vi "纳清电导率电极校准.vi"() -> ()   [LabVIEW 2016, in "斯坦道多参数.lvlib"]
uses:
  <vilib>/Utility/miscctls.llb/LVPointTypeDef.ctl
  <vilib>/Utility/miscctls.llb/LVPositionTypeDef.ctl
  <vilib>/Analysis/NI_AALBase.lvlib
panel:
  out "当前量程":u16
  out "当前探头类别":string
  out "报警信息":string
  out "温度校准参数":sgl format="%#.2f"
  out "通讯状态":string
  out "第二点校准值":dbl
  out "第一点校准值":dbl
  in  "校准停止":bool
  in  "校准启动":bool
  in  "校准模式":enum16{"单点校准"}(ring)
  out "最小值":sgl format="%#.2f"
  out "最大值":sgl format="%#.2f"
  out "波形图表":sgl(graph) caption="历史曲线"
  out "mean":dbl caption="均值" format="%#.2f"
  out "standard deviation":dbl caption="标准差" format="%#.2f"
  out "变异系数":dbl format="%#.6f"
  out "测量值":sgl format="%#.2f"
  out "提示":string
  out "标液1":sgl
  out "原始光强数值":sgl caption="信号值" format="%#.6f"
  out "温度":dbl format="%#.2f"
  # "电导率电极设定"
  # "℃"
  # "uS/cm"
  # "电阻"
  # "℃"
  # "请选择校准模式:"
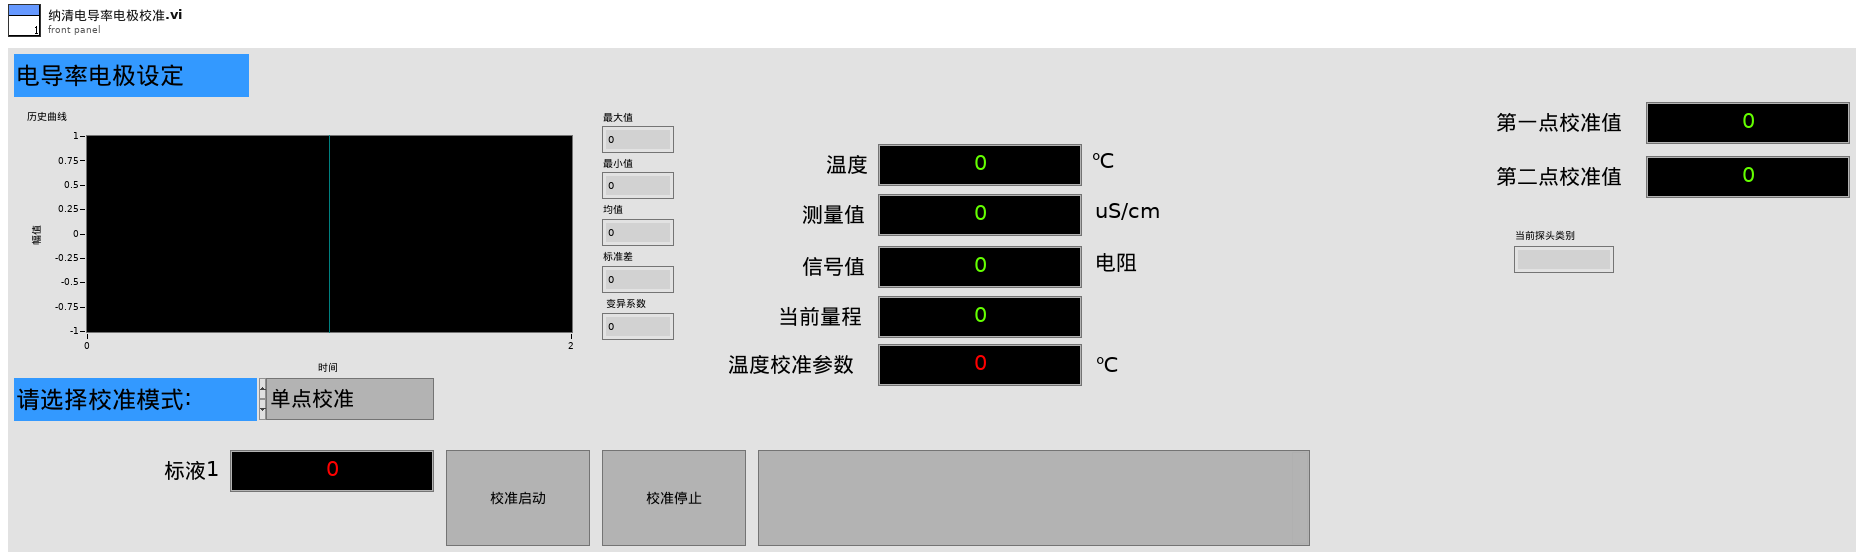
[diagram p1: front panel]
types:
  T1 = typedef "LVPointTypeDef.ctl" = cluster{"Horizontal":i16, "Vertical":i16}
  T2 = typedef "斯坦道多参数.lvlib/校准步骤.ctl" = enum16{"待机", "放置第一点标液", "第一点校准启动", "第一点校准写入", "第一点校准失败", "放置第二点标液", "第二点校准启动", "第二点校准写入", "第二点校准失败", "放置第三点标液", "第三点校准启动", "第三点校准写入", "第三点校准失败", "校准结果写入", "校准结束"}
  T3 = cluster{"报警码":u16, "电导率数据（uS/cm）":sgl, "0x0003 NC":sgl, "温度数据":sgl, "电导率原始信号电阻":sgl, "当前量程":u16, "温度补偿系数":sgl, "0X0009_NC":string, "产品名称":string, "序列号":string, "硬件版本":string, "软件版本":string, "通讯地址":u16, "波特率":u16, "设备类型":u16, "0X0026_NC":string, "第一点原始数据":sgl, "第一点校准数据":sgl, "0X0035_NC":sgl, "0X0037_NC":sgl, "探头校准命令":u16, "温度校准参数":sgl, "温度校准命令":u16}
  T4 = typedef "LVPositionTypeDef.ctl" = cluster{"Left":i32, "Top":i32}
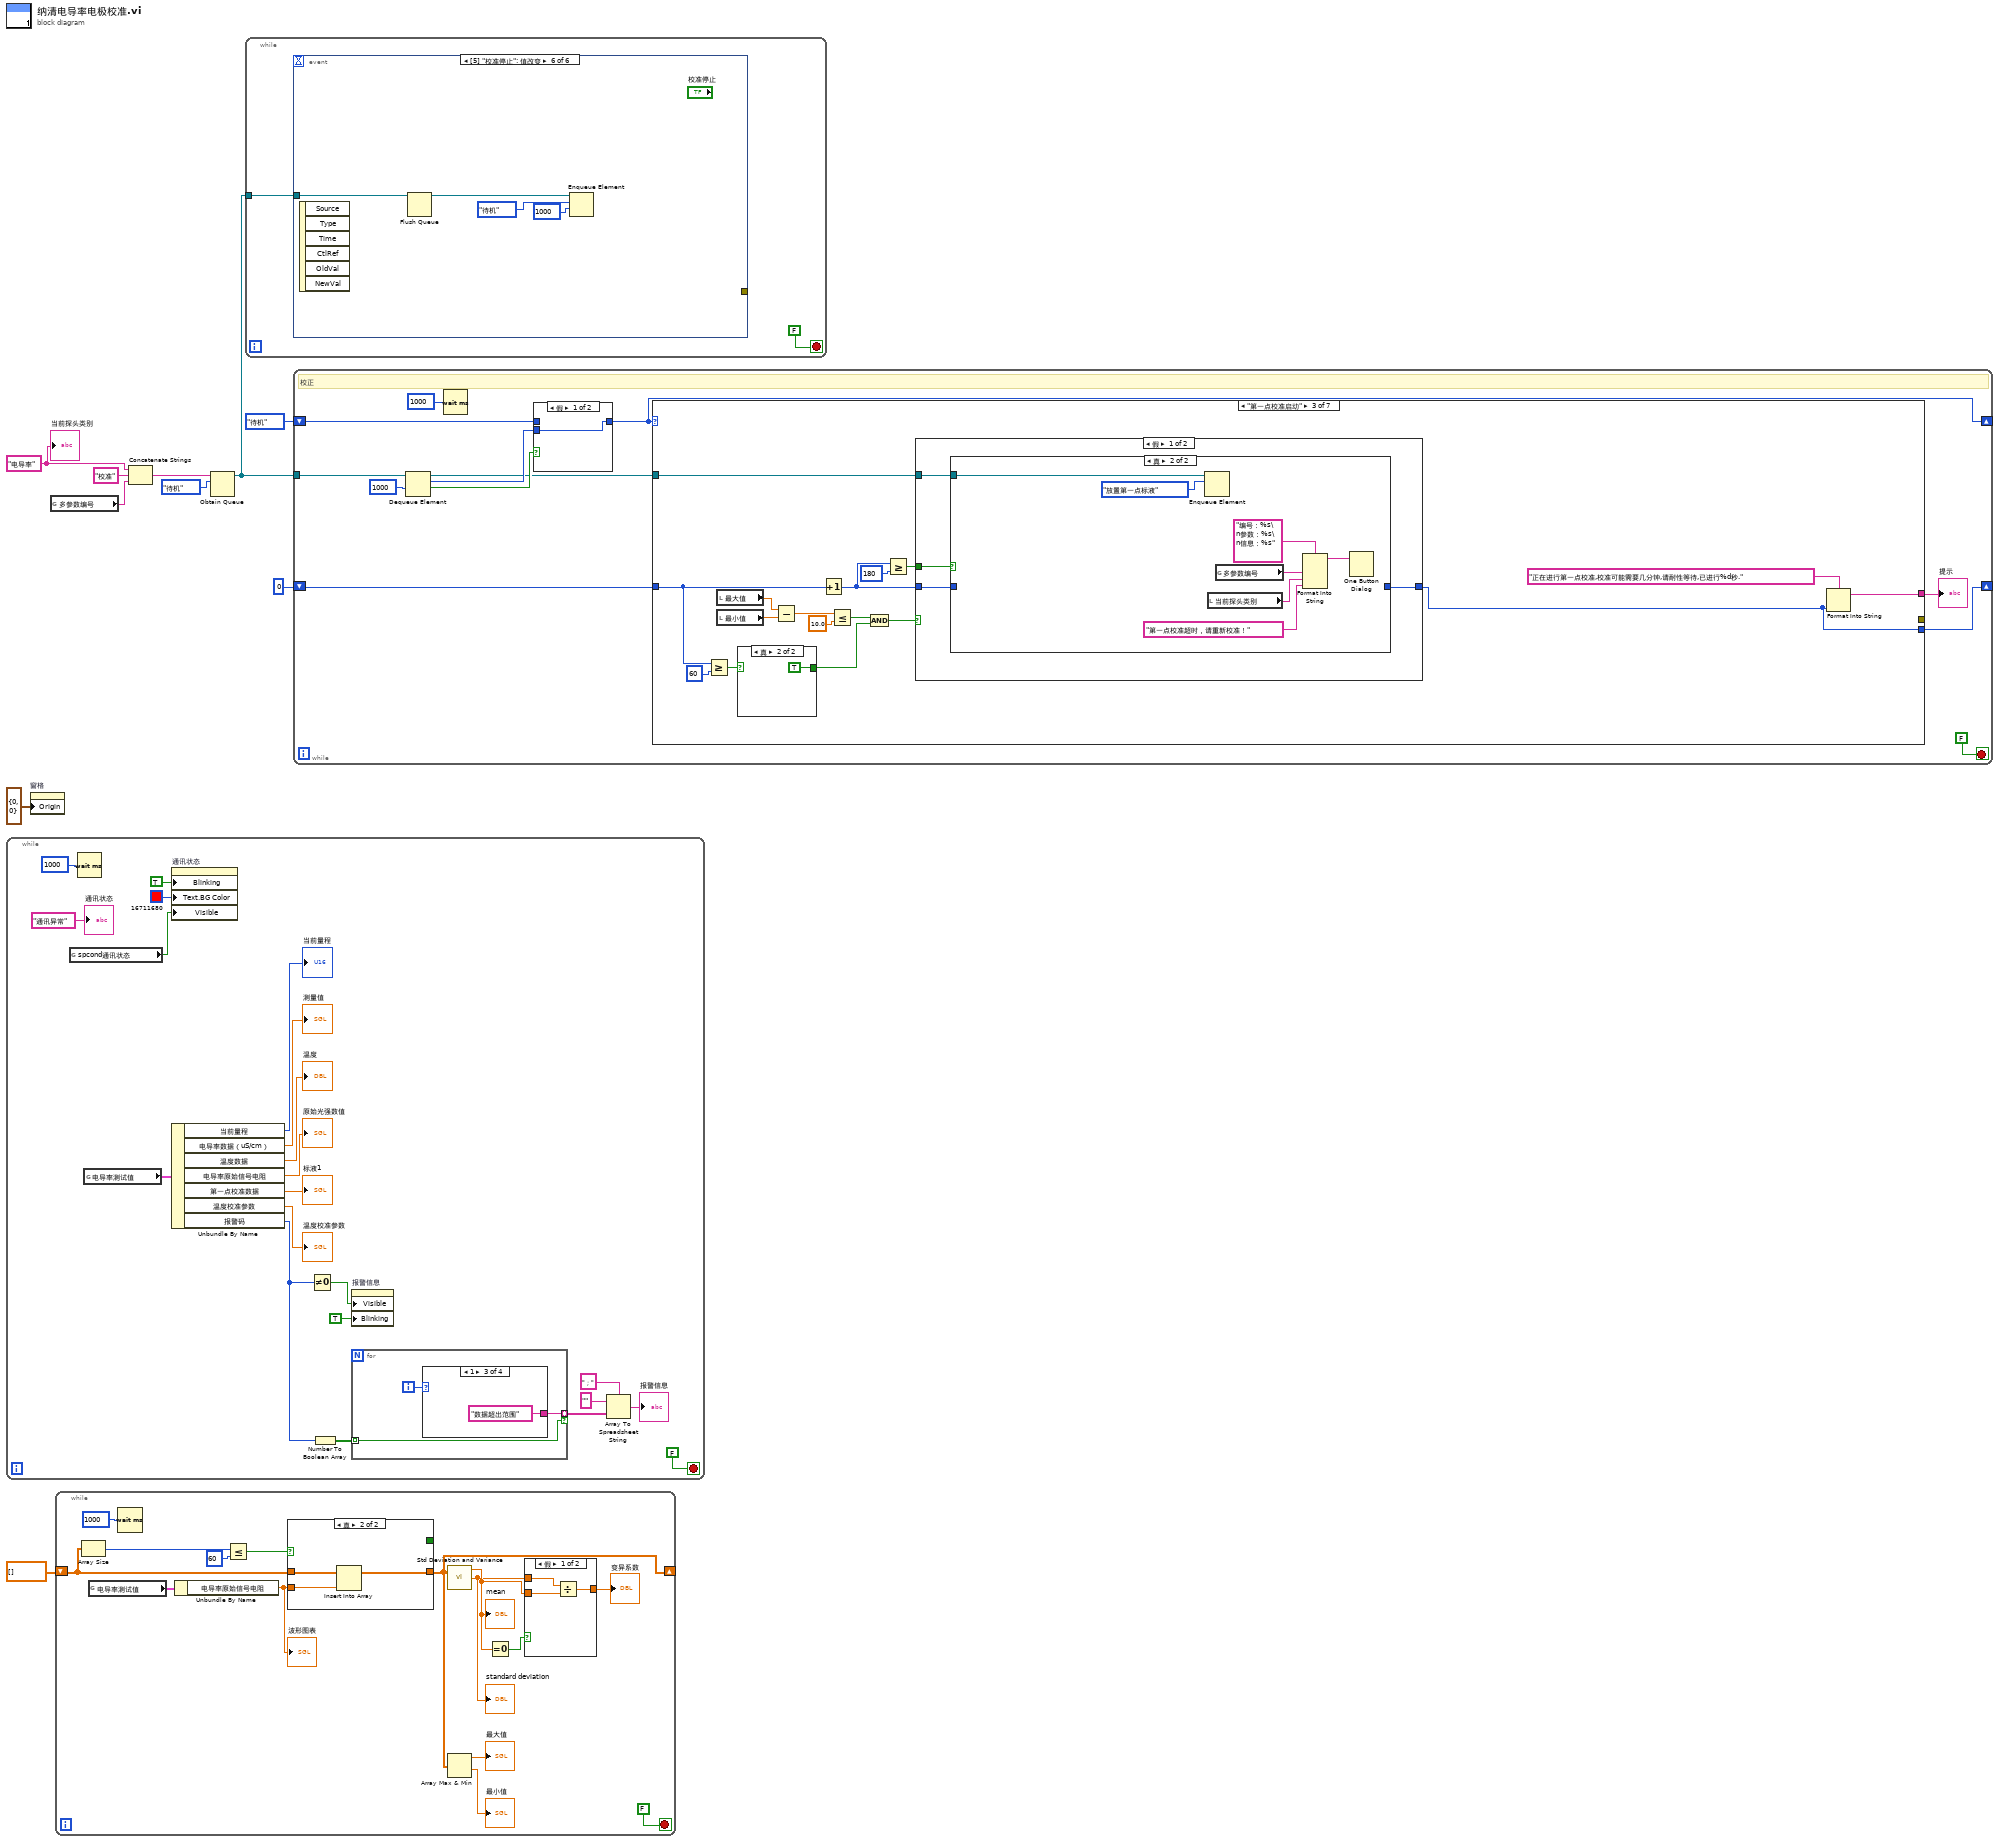
[diagram p0: block diagram]
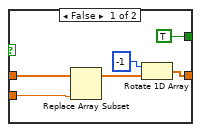
[diagram p3: hidden frame]
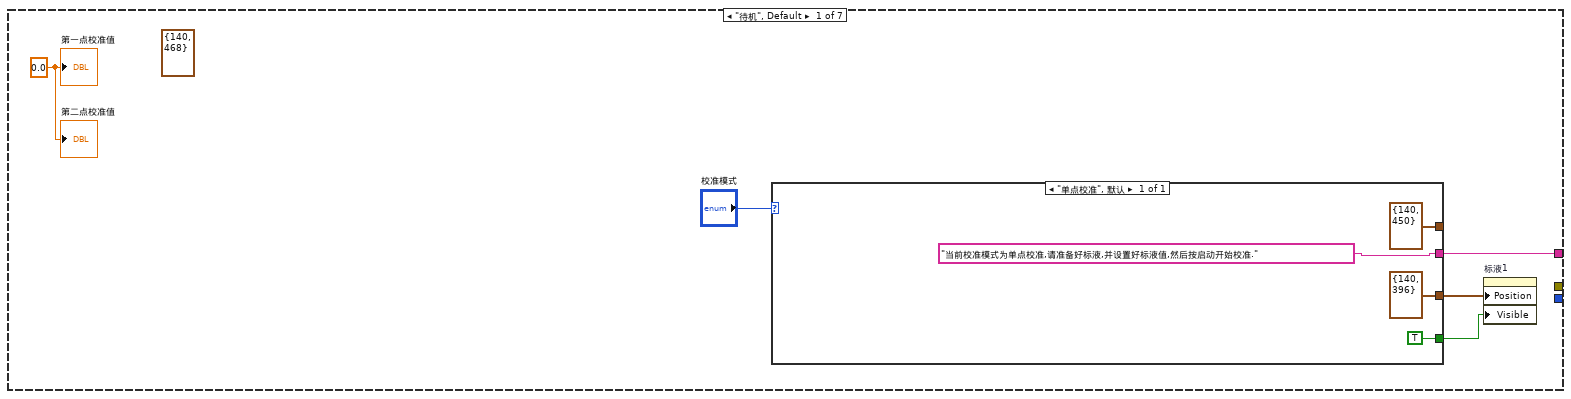
[diagram p5: hidden frame]
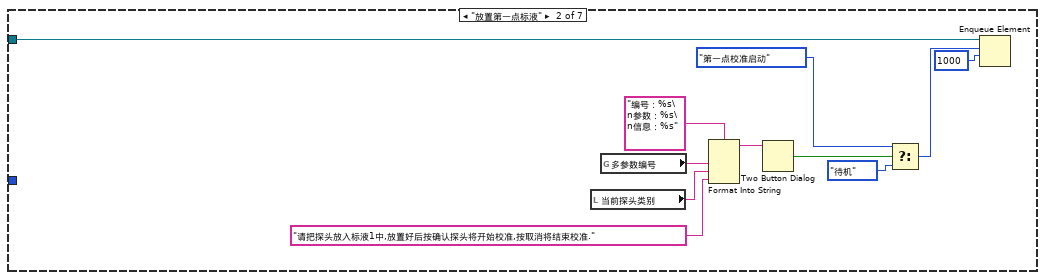
[diagram p6: hidden frame]
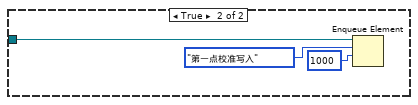
[diagram p8: hidden frame]
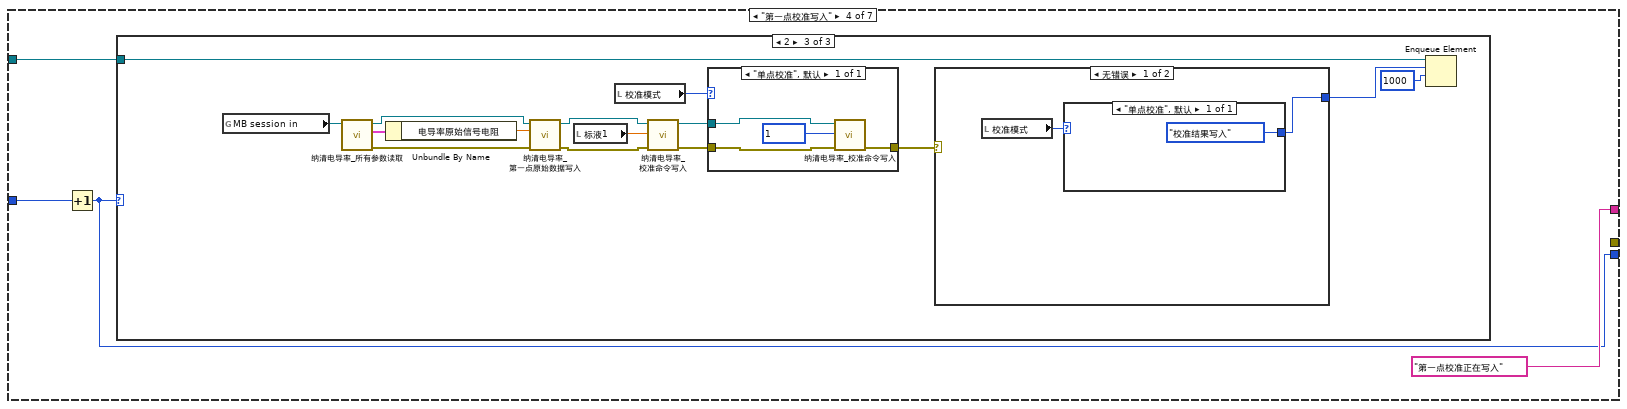
[diagram p10: hidden frame]
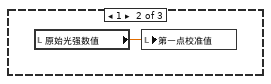
[diagram p12: hidden frame]
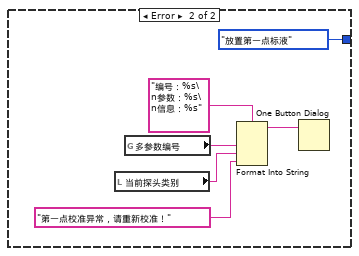
[diagram p13: hidden frame]
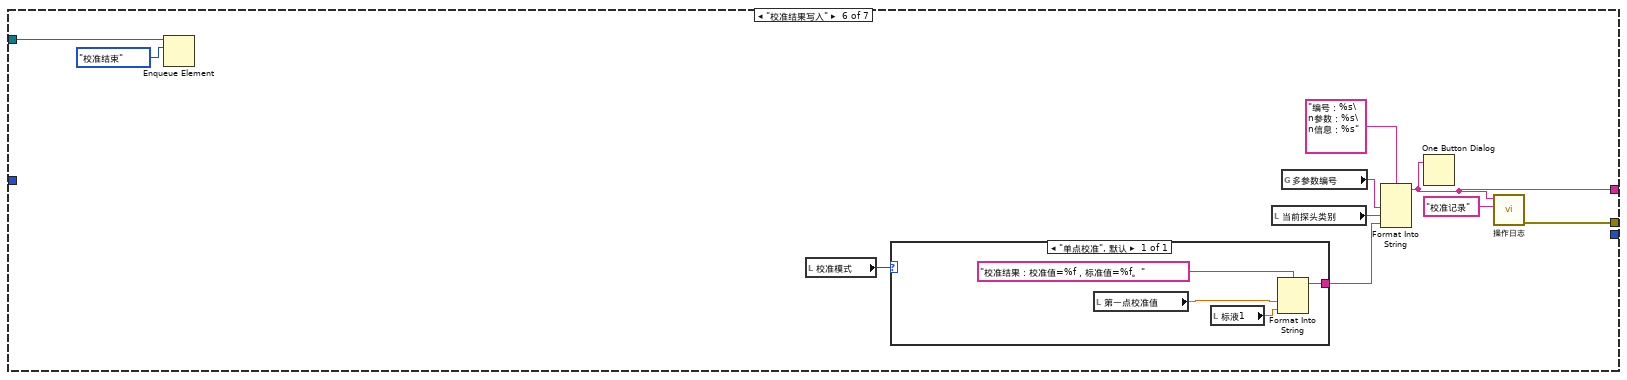
[diagram p15: hidden frame]
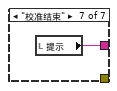
[diagram p16: hidden frame]
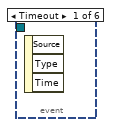
[diagram p17: hidden frame]
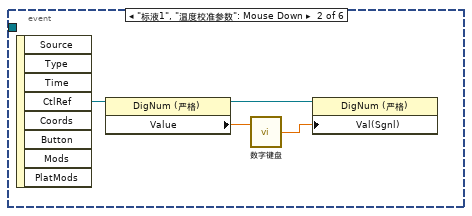
[diagram p18: hidden frame]
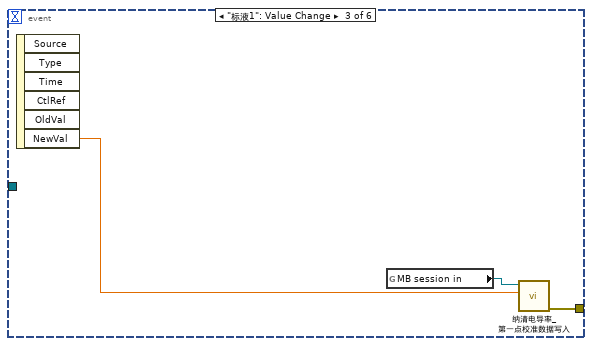
[diagram p19: hidden frame]
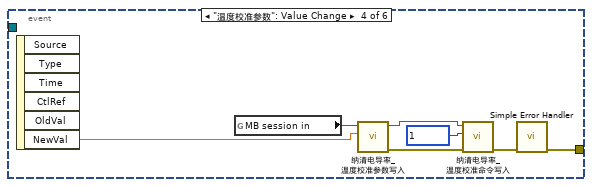
[diagram p20: hidden frame]
diagram:
  w1 = "电导率" ("当前探头类别")
  n1 = while {
    stop <- FALSE stop-if-true
    n2 = global read "多参数全局变量.vi" "spcond通讯状态"() -> (w21:bool)
    n3 = Wait (ms)(milliseconds to wait=u32 1000 ("等待时间（毫秒）")) -> ()  [unwired: 1 out]
    n4 = global read "纳清过程全局变量.vi" "电导率测试值"() -> (w29:T3)
    n5 = property on="通讯状态" class="Str"("Blinking"=TRUE ("闪烁"), "Text.BG Color"=u32 16711680, "Visible"=w21) -> ()  [unwired: 2 in, 2 out]
    n6 = Unbundle By Name(w29) -> ("当前量程"=→"当前量程":u16, "电导率数据（uS/cm）"=→"测量值":sgl, "温度数据"=→"温度":sgl, "电导率原始信号电阻"=→"原始光强数值":sgl, "第一点校准数据"=→"标液1":sgl, "温度校准参数"=→"温度校准参数":sgl, "报警码"=w14:u16)
    n7 = Not Equal To 0?(x=w14) -> (x != 0?=w13:bool)
    n8 = Number To Boolean Array(number=w14) -> (Boolean array=w19:bool[])
    n9 = property on="报警信息" class="Str"("Visible"=w13, "Blinking"=TRUE ("闪烁")) -> ()  [unwired: 2 in, 2 out]
    n10 = for {
      tunnel: w19 -> [w32] mode=indexing
      tunnel: [w33] -> w18 mode=indexing if=w32
      i -> [w34]
      n11 = case shown="1" w34 {
        tunnel: [_ "温度超出范围" "数据超出范围" "温度传感器故障"] -> w33
        frame Default {
        }
        frame 0 {
        }
        frame 1 {
        }
        frame 8 {
        }
      }
    }
    n12 = Array To Spreadsheet String(delimiter (Tab)="；" ("分隔符(Tab)"), array=w18, 3:"" ("格式字符串")) -> (spreadsheet string=→"报警信息":string)
    "通讯状态" <- "通讯异常" ("当前串口")
  }
  n13 = property on="窗格" class="Pane"("Origin"=T1 {"Horizontal"=0, "Vertical"=0} ("原点")) -> ()  [unwired: 2 in, 2 out]
  n14 = global read "多参数全局变量.vi" "多参数编号"() -> (w2:string)
  n15 = while {
    shift-right: [w42] -> _
    shift-left: sgl[] [] -> [w48]
    stop <- FALSE stop-if-true
    n16 = Array Size(array=w48) -> (size(s)=w50:i32)
    n17 = global read "纳清过程全局变量.vi" "电导率测试值"() -> (w38:T3)
    n18 = Wait (ms)(milliseconds to wait=u32 1000 ("等待时间（毫秒）")) -> ()  [unwired: 1 out]
    n19 = Unbundle By Name(w38) -> ("电导率原始信号电阻"=w39:sgl)
    "波形图表" <- w39
    n20 = Less Or Equal?(x=w50, y=60) -> (x <= y?=w49:bool)
    n21 = case shown="真" w49 {
      tunnel: w48 -> [w61 w64]
      tunnel: w39 -> [w59 w63]
      tunnel: [w57 w62] -> w42
      tunnel: [TRUE _] -> _
      frame False {
        n22 = Replace Array Subset(array=w61, new element=w59) -> (w60:sgl[])  [unwired: 1 in]
        n23 = Rotate 1D Array(1:w60, 2:-1 ("n")) -> (0:w57:sgl[])
      }
      frame True {
        n24 = Insert Into Array(array=w64, new element=w63) -> (w62:sgl[])  [unwired: 1 in]
      }
    }
    n25 = call <vilib>:"Std Deviation and Variance.vi"("X"=w42) -> ("mean"=w46:dbl, "standard deviation"=w45:dbl)  [unwired: 1 in, 1 out]
    "mean" <- w46
    "standard deviation" <- w45
    n26 = Array Max & Min(array=w42) -> (max value=→"最大值":sgl, min value=→"最小值":sgl)  [unwired: 2 out]
    n27 = Equal To 0?(x=w46) -> (x = 0?=w47:bool)
    n28 = case shown="假" w47 {
      tunnel: w45 -> [w55 _]
      tunnel: [w54 _] -> w44
      tunnel: w46 -> [w53 _]
      frame False {
        n29 = Divide(x=w55, y=w53) -> (x/y=w54:dbl)
      }
      frame True {
      }
    }
    "变异系数" <- w44
  }
  n30 = Concatenate Strings(w1, "校准" ("名称（未命名）"), w2) -> (w3:string)
  n31 = Obtain Queue(name (unnamed)=w3, element data type=校准步骤."待机" ("枚举")) -> (queue out=w5:refnum<queue>)  [unwired: 3 in, 2 out]
  n32 = while {
    tunnel: w5 -> [w65]
    stop <- FALSE stop-if-true
    n33 = event shown="[5] \"校准停止\": 值改变" {
      selector: _ -> [_ _ _ _ _ _]
      dyn-events: _ -> [_ _ _ _ _ _]
      timeout: _ -> [_ _ _ _ _ _]
      tunnel: [_ _ w72 w74 _ _] -> _
      tunnel: w65 -> [_ _ _ _ w81 w83]
      event Timeout {
        n34 = event-data() -> ()  [unwired: 1 in, 3 out]
      }
      event "标液1", "温度校准参数": Mouse Down {
        n35 = event-data() -> ("CtlRef"=w67:refnum<vi>)  [unwired: 1 in, 7 out]
        n36 = property class="DigNum (严格)"(reference=w67) -> (reference out=w68:refnum<vi>, "Value"=w69:sgl)  [unwired: 1 in, 1 out]
        n37 = call "数字键盘.vi"("OldNumber"=w69) -> ("NewNumber"=w70:dbl)  [unwired: 1 in]
        n38 = property class="DigNum (严格)"(reference=w68, "Val(Sgnl)"=w70) -> ()  [unwired: 1 in, 2 out]
      }
      event "标液1": Value Change {
        n39 = event-data() -> ("NewVal"=w71:sgl)  [unwired: 1 in, 5 out]
        n40 = global read "多参数全局变量.vi" "MB session in"() -> (w73:refnum<class "MB_Master.lvclass">)
        n41 = call "纳清电导率_第一点校准数据写入.vi"("数值"=w71, "MB session in"=w73) -> ("error out"=w72:errorcluster)  [unwired: 8 in, 1 out]
      }
      event "温度校准参数": Value Change {
        n42 = event-data() -> ("NewVal"=w79:sgl)  [unwired: 1 in, 5 out]
        n43 = global read "多参数全局变量.vi" "MB session in"() -> (w78:refnum<class "MB_Master.lvclass">)
        n44 = call "纳清电导率_温度校准参数写入.vi"("数值"=w79, "MB session in"=w78) -> ("error out"=w80:errorcluster, "MB session out"=w77:refnum<class "MB_Master.lvclass">)  [unwired: 8 in]
        n45 = call "纳清电导率_温度校准命令写入.vi"("error in (no error)"=w80, "数值"=u16 1 ("starting address"), "MB session in"=w77) -> ("error out"=w75:errorcluster)  [unwired: 7 in, 1 out]
        n46 = call <vilib>:"Simple Error Handler.vi"("error in (no error)"=w75) -> ("error out"=w74:errorcluster)  [unwired: 4 in, 4 out]
      }
      event "校准启动": Value Change {
        n47 = event-data() -> ()  [unwired: 1 in, 6 out]
        n48 = Enqueue Element(queue=w81, element=校准步骤."放置第一点标液" ("元素")) -> ()  [unwired: 2 in, 3 out]
      }
      event "校准停止": Value Change {
        n49 = event-data() -> ()  [unwired: 1 in, 6 out]
        n50 = Flush Queue(queue=w83) -> (queue out=w84:refnum<queue>)  [unwired: 1 in, 2 out]
        n51 = Enqueue Element(queue=w84, element=校准步骤."待机" ("元素"), timeout in ms (-1)=1000 ("超时毫秒(-1)")) -> ()  [unwired: 1 in, 3 out]
      }
    }
  }
  n52 = while "While循环" {
    shift-right: [w88] -> _
    shift-left: 校准步骤."待机" ("枚举") -> [w90]
    shift-right: [w87] -> _
    shift-left: 0 -> [w96]
    tunnel: w5 -> [w91]
    stop <- FALSE stop-if-true
    # "校正"
    n53 = Dequeue Element(queue=w91, timeout in ms (-1)=1000 ("超时毫秒(-1)")) -> (queue out=w89:refnum<queue>, element=w92:T2, timed out?=w93:bool)  [unwired: 1 in, 1 out]
    n54 = Wait (ms)(milliseconds to wait=u32 1000 ("等待时间（毫秒）")) -> ()  [unwired: 1 out]
    n55 = case shown="假" w93 {
      tunnel: w92 -> [w99 _]
      tunnel: [w99 w100] -> w88
      tunnel: w90 -> [_ w100]
      frame False {
      }
      frame True {
      }
    }
    n56 = case shown="\"第一点校准启动\"" w88 {
      tunnel: [w104 _ w122 "第一点校准正在写入" ("提示") _ w189 w201] -> w95
      tunnel: w96 -> [_ _ w123 w156 _ _ _]
      tunnel: [_ _ w121 w154 _ _ _] -> w87
      tunnel: w89 -> [_ w116 w124 w155 _ w195 _]
      tunnel: [_ _ _ _ _ w193 _] -> _
      frame "待机", Default {
        (unwired) T4 {"Left"=140, "Top"=468} ("位置 3")
        w101 = 0.0 ("第一点校准值")
        n57 = case shown="\"单点校准\", 默认" "校准模式" {
          tunnel: ["当前校准模式为单点校准,请准备好标液,并设置好标液值,然后按启动开始校准." ("提示")] -> w104
          tunnel: [T4 {"Left"=140, "Top"=396} ("位置")] -> w103
          tunnel: [T4 {"Left"=140, "Top"=450} ("位置 2")] -> _
          tunnel: [TRUE ("可见")] -> w102
          frame "单点校准", Default {
          }
        }
        n58 = property on="标液1" class="DigNum (严格)"("Position"=w103, "Visible"=w102) -> ()  [unwired: 2 in, 2 out]
        "第一点校准值" <- w101
        "第二点校准值" <- w101
      }
      frame "放置第一点标液" {
        n59 = local read "当前探头类别"() -> (w110:string)
        n60 = global read "多参数全局变量.vi" "多参数编号"() -> (w114:string)
        n61 = Format Into String(format string="编号：%s\n参数：%s\n信息：%s" ("格式字符串"), w114, w110, "请把探头放入标液1中,放置好后按确认探头将开始校准,按取消将结束校准." ("消息")) -> (resulting string=w113:string)  [unwired: 2 in, 1 out]
        n62 = Two Button Dialog(message=w113) -> (T button?=w111:bool)  [unwired: 2 in]
        n63 = Select(t=校准步骤."第一点校准启动" ("元素"), s=w111, f=校准步骤."待机" ("元素")) -> (s? t:f=w117:T2)
        n64 = Enqueue Element(queue=w116, element=w117, timeout in ms (-1)=1000 ("超时毫秒(-1)")) -> ()  [unwired: 1 in, 3 out]
      }
      frame "第一点校准启动" {
        n65 = Greater Or Equal?(x=w123, y=60) -> (x >= y?=w130:bool)
        n66 = local read "最大值"() -> (w133:sgl)
        n67 = local read "最小值"() -> (w132:sgl)
        n68 = case shown="真" w130 {
          tunnel: [_ TRUE] -> w131
          frame False {
          }
          frame True {
          }
        }
        n69 = Subtract(x=w133, y=w132) -> (x-y=w134:sgl)
        n70 = Increment(x=w123) -> (x+1=w137:i32)
        n71 = Less Or Equal?(x=w134, y=10.0) -> (x <= y?=w127:bool)
        n72 = And(x=w127, y=w131) -> (x .and. y?=w135:bool)
        n73 = Greater Or Equal?(x=w137, y=180) -> (x >= y?=w136:bool)
        n74 = case shown="假" w135 {
          tunnel: w124 -> [w140 w152]
          tunnel: w136 -> [w141 _]
          tunnel: w137 -> [w139 _]
          tunnel: [w138 _] -> w121
          frame False {
            n75 = case shown="真" w141 {
              tunnel: w140 -> [_ w149]
              tunnel: w139 -> [w142 _]
              tunnel: [w142 _] -> w138
              frame False {
              }
              frame True {
                n76 = Enqueue Element(queue=w149, element=校准步骤."放置第一点标液" ("元素")) -> ()  [unwired: 2 in, 3 out]
                n77 = local read "当前探头类别"() -> (w143:string)
                n78 = global read "多参数全局变量.vi" "多参数编号"() -> (w146:string)
                n79 = Format Into String(format string="编号：%s\n参数：%s\n信息：%s" ("格式字符串"), w146, w143, "第一点校准超时，请重新校准！" ("error source (\" \")")) -> (resulting string=w144:string)  [unwired: 2 in, 1 out]
                n80 = One Button Dialog(message=w144) -> ()  [unwired: 1 in, 1 out]
              }
            }
          }
          frame True {
            n81 = Enqueue Element(queue=w152, element=校准步骤."第一点校准写入" ("元素"), timeout in ms (-1)=1000 ("超时毫秒(-1)")) -> ()  [unwired: 1 in, 3 out]
          }
        }
        n82 = Format Into String(format string="正在进行第一点校准,校准可能需要几分钟,请耐性等待,已进行%d秒." ("格式字符串"), w121) -> (resulting string=w122:string)  [unwired: 2 in, 1 out]
      }
      frame "第一点校准写入" {
        n83 = Increment(x=w156) -> (x+1=w154:i32)
        n84 = case shown="2" w154 {
          tunnel: w155 -> [_ _ w173]
          frame 0, Default {
          }
          frame 1 {
            n85 = local read "原始光强数值"() -> (w158:sgl)
            n86 = local write "第一点校准值"(w158) -> ()
          }
          frame 2 {
            n87 = global read "多参数全局变量.vi" "MB session in"() -> (w169:refnum<class "MB_Master.lvclass">)
            n88 = call "纳清电导率_所有参数读取.vi"("MB session in"=w169) -> ("error out"=w171:errorcluster, "输出值"=w168:T3, "MB session out"=w170:refnum<class "MB_Master.lvclass">)  [unwired: 8 in]
            n89 = Unbundle By Name(w168) -> ("电导率原始信号电阻"=w167:sgl)
            n90 = call "纳清电导率_第一点原始数据写入.vi"("error in (no error)"=w171, "数值"=w167, "MB session in"=w170) -> ("error out"=w166:errorcluster, "MB session out"=w165:refnum<class "MB_Master.lvclass">)  [unwired: 7 in]
            n91 = local read "标液1"() -> (w162:sgl)
            n92 = local read "校准模式"() -> (w159:enum16{"单点校准"})
            n93 = call "纳清电导率_校准命令写入.vi"("error in (no error)"=w166, "数值"=w162, "MB session in"=w165) -> ("error out"=w164:errorcluster, "MB session out"=w163:refnum<class "MB_Master.lvclass">)  [unwired: 7 in]
            n94 = case shown="\"单点校准\", 默认" w159 {
              tunnel: w164 -> [w177]
              tunnel: w163 -> [w176]
              tunnel: [w174] -> w161
              frame "单点校准", Default {
                n95 = call "纳清电导率_校准命令写入.vi"("error in (no error)"=w177, "数值"=u16 1 ("starting address"), "MB session in"=w176) -> ("error out"=w174:errorcluster)  [unwired: 7 in, 1 out]
              }
            }
            n96 = case shown="无错误" w161 {
              tunnel: [w178 校准步骤."放置第一点标液" ("元素")] -> w160
              frame No Error {
                n97 = local read "校准模式"() -> (w179:enum16{"单点校准"})
                n98 = case shown="\"单点校准\", 默认" w179 {
                  tunnel: [校准步骤."校准结果写入" ("元素")] -> w178
                  frame "单点校准", Default {
                  }
                }
              }
              frame Error {
                n99 = local read "当前探头类别"() -> (w181:string)
                n100 = global read "多参数全局变量.vi" "多参数编号"() -> (w185:string)
                n101 = Format Into String(format string="编号：%s\n参数：%s\n信息：%s" ("格式字符串"), w185, w181, "第一点校准异常，请重新校准！" ("error source (\" \")")) -> (resulting string=w183:string)  [unwired: 2 in, 1 out]
                n102 = One Button Dialog(message=w183) -> ()  [unwired: 1 in, 1 out]
              }
            }
            n103 = Enqueue Element(queue=w173, element=w160, timeout in ms (-1)=1000 ("超时毫秒(-1)")) -> ()  [unwired: 1 in, 3 out]
          }
        }
      }
      frame "第一点校准失败" {
      }
      frame "校准结果写入" {
        n104 = Enqueue Element(queue=w195, element=校准步骤."校准结束" ("元素")) -> ()  [unwired: 2 in, 3 out]
        n105 = local read "校准模式"() -> (w194:enum16{"单点校准"})
        n106 = case shown="\"单点校准\", 默认" w194 {
          tunnel: [w200] -> w190
          frame "单点校准", Default {
            n107 = local read "第一点校准值"() -> (w199:dbl)
            n108 = local read "标液1"() -> (w197:sgl)
            n109 = Format Into String(format string="校准结果：校准值=%f，标准值=%f。" ("提示"), w199, w197) -> (resulting string=w200:string)  [unwired: 2 in, 1 out]
          }
        }
        n110 = local read "当前探头类别"() -> (w187:string)
        n111 = global read "多参数全局变量.vi" "多参数编号"() -> (w191:string)
        n112 = Format Into String(format string="编号：%s\n参数：%s\n信息：%s" ("格式字符串"), w191, w187, w190) -> (resulting string=w189:string)  [unwired: 2 in, 1 out]
        n113 = One Button Dialog(message=w189) -> ()  [unwired: 1 in, 1 out]
        n114 = call "操作日志.vi"("table"="校准记录", "日志信息"=w189) -> ("error out"=w193:errorcluster)  [unwired: 9 in]
      }
      frame "校准结束" {
        n115 = local read "提示"() -> (w201:string)
      }
    }
    "提示" <- w95
  }
  "当前探头类别" <- w1
